vi "Cancel_Prompt.vi"(3 "error in (no error)":errorcluster) -> (0 "error out":errorcluster, 1 "Enum 2":enum16{"Unload Lot", "Unload and delete data"}(ring), 2 "Cancelled?":bool)   [LabVIEW 2012]
doc: "Use this template to create a dialog box with event handling."
panel:
  in  "Enum":enum16{"Unload Lot", "Unload and delete data"}(ring)
  in  "Cancel":bool
  in  "OK":bool
  # "What would you like to do?\n\nUnload Lot:  Enables New/Load Buttons\nUnload and Delete data:\nDeletes Data  on Database and \nEnables New/Load Buttons\n** WARNING ** CANNOT BE UNDONE"
  # "Select Option"
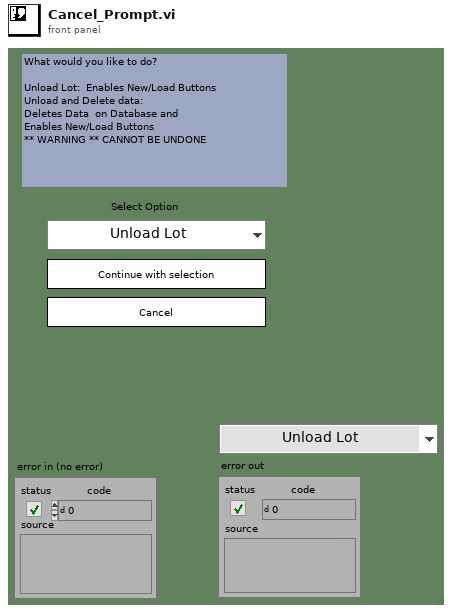
[diagram p1: front panel]
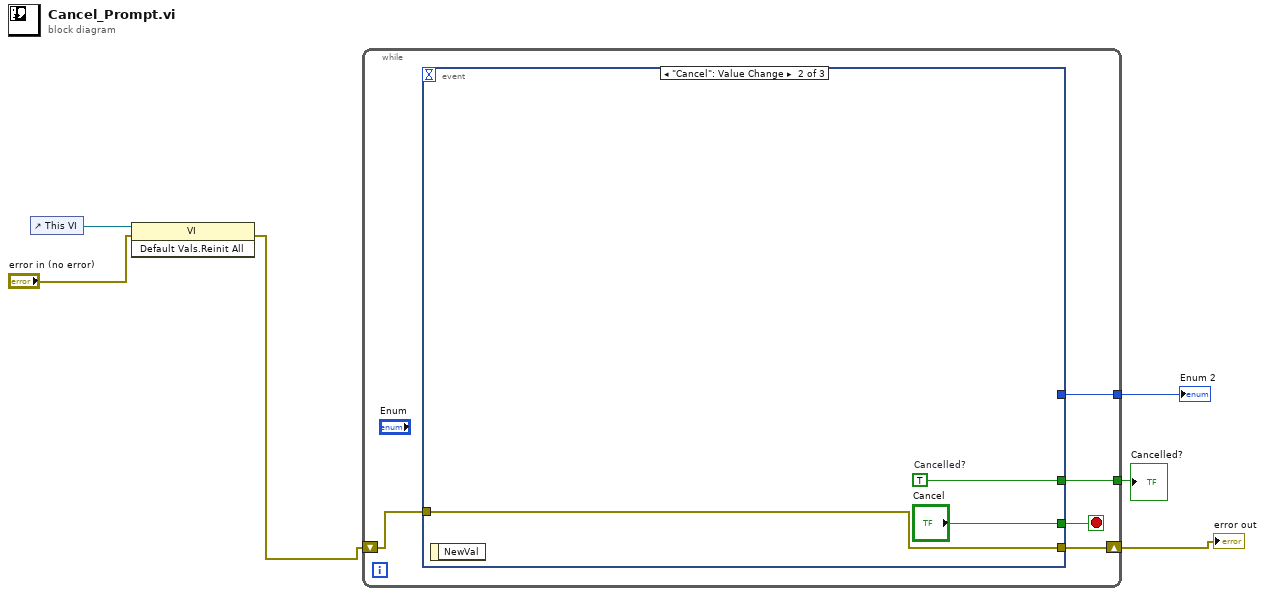
[diagram p0: block diagram]
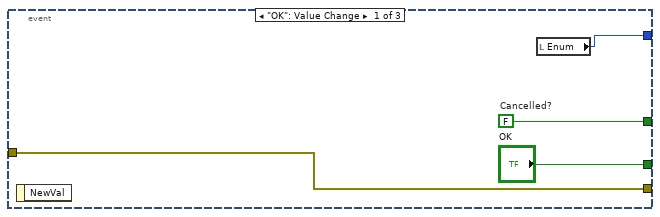
[diagram p2: hidden frame]
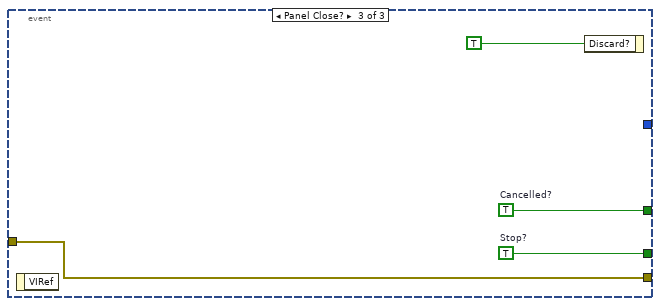
[diagram p3: hidden frame]
diagram:
  n1 = control-ref of="This VI"() -> (w3:refnum<vi>)
  n2 = invoke class="VI" method="Default Vals.Reinit All"(reference=w3, error in="error in (no error)") -> (error out=w1:errorcluster)  [unwired: 1 in, 2 out]
  n3 = while {
    tunnel: [w10] -> w6
    tunnel: [w9] -> w5
    shift-right: [w8] -> w4
    shift-left: w1 -> [w7]
    stop <- w11 stop-if-true
    n4 = event shown="[1] \"Cancel\": Value Change" {
      selector: _ -> [_ _ _]
      dyn-events: _ -> [_ _ _]
      timeout: _ -> [_ _ _]
      tunnel: ["OK" "Cancel" w21] -> w11
      tunnel: [w15 w18 w20] -> w10
      tunnel: [w13 _ _] -> w9
      tunnel: [w12 w16 w19] -> w8
      tunnel: w7 -> [w12 w16 w19]
      event "OK": Value Change {
        w15 = FALSE  # Cancelled?
        n5 = event-data() -> ()  [unwired: 1 in, 1 out]
        n6 = local read "Enum"() -> (w13:enum16{"Unload Lot", "Unload and delete data"})
      }
      event "Cancel": Value Change {
        w18 = TRUE  # Cancelled?
        n7 = event-data() -> ()  [unwired: 1 in, 1 out]
      }
      event Panel Close? {
        w20 = TRUE  # Cancelled?
        w21 = TRUE  # Stop?
        n8 = event-data() -> ()  [unwired: 1 in, 1 out]
        n9 = event-data("Discard?"=TRUE) -> ()  [unwired: 1 in, 1 out]
      }
    }
  }
  "Cancelled?" <- w6
  "Enum 2" <- w5
  "error out" <- w4
